vi "5子棋.vi"() -> ()   [LabVIEW 2014]
uses:
  <vilib>/Utility/miscctls.llb/LVPositionTypeDef.ctl
panel:
  out "Black":bool[][](array[boolean])
  out "White":bool[][](array[boolean])
  in  "新遊戲":bool
  out "步數":i32
  in  "結束":bool
  out "悔棋":bool
  out "black control":bool[][](array[boolean])
  out "white control":bool[][](array[boolean])
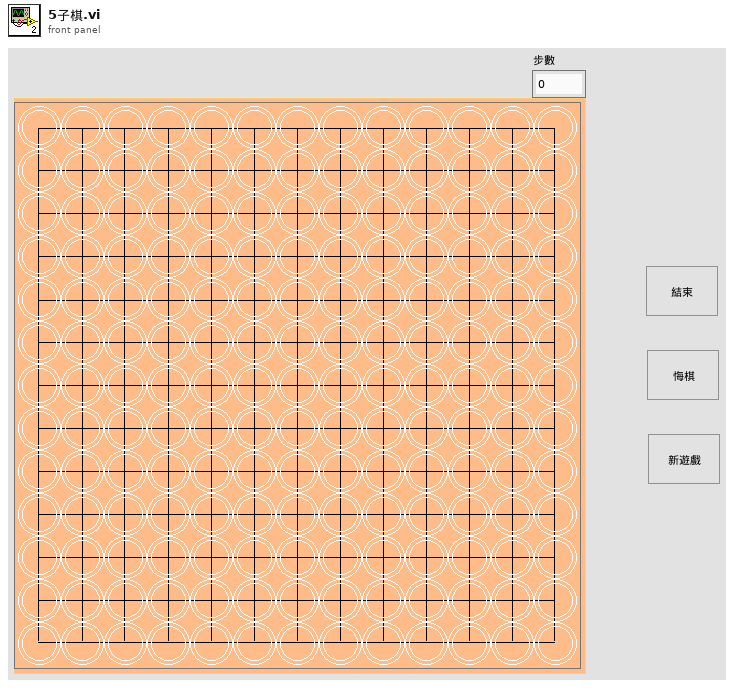
[diagram p1: front panel]
types:
  T1 = typedef "LVPositionTypeDef.ctl" = cluster{"Left":i32, "Top":i32}
  T2 = typedef "LVPoint32TypeDef.ctl" = cluster{"Horizontal":i32, "Vertical":i32}
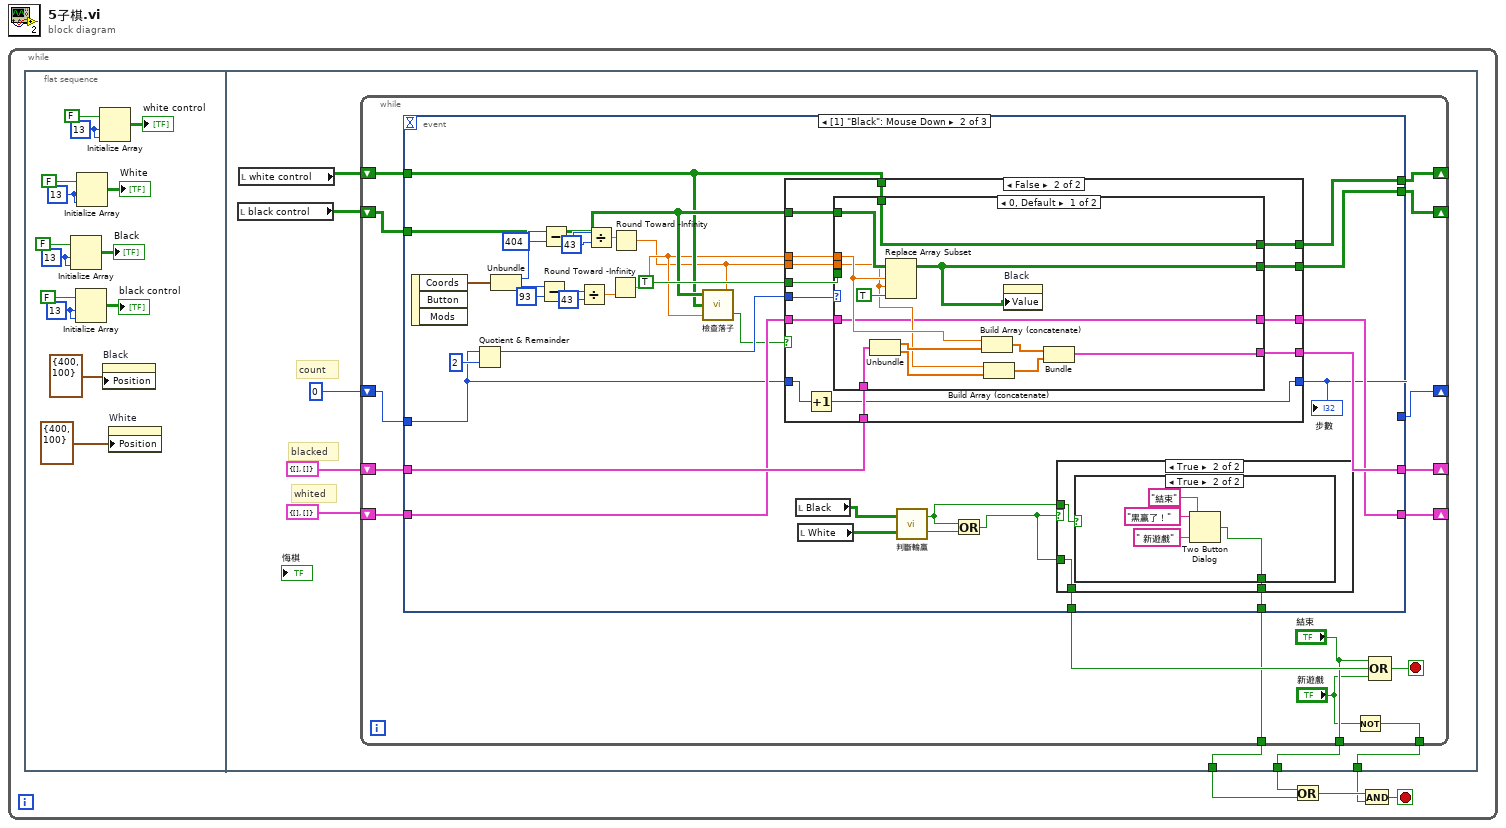
[diagram p0: block diagram]
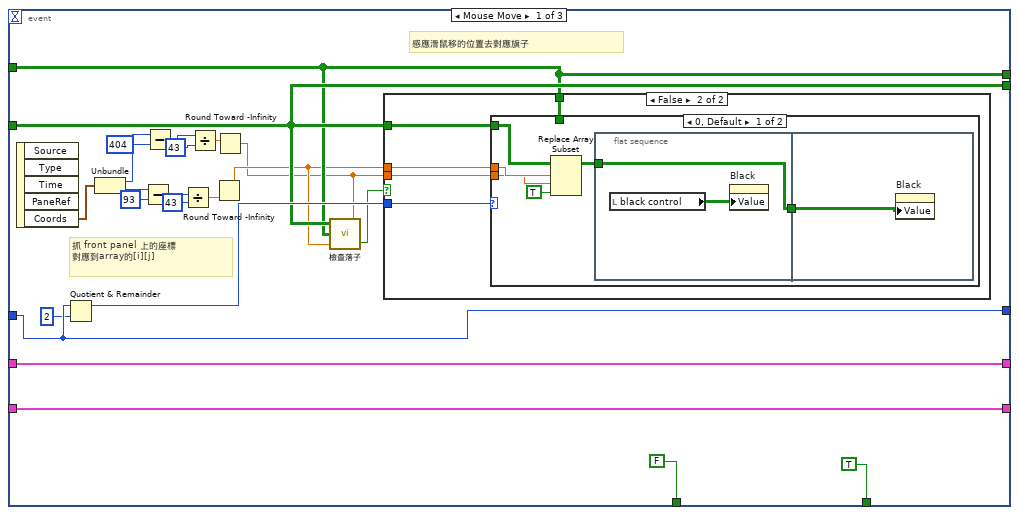
[diagram p2: hidden frame]
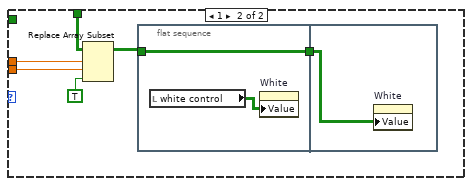
[diagram p4: hidden frame]
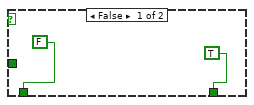
[diagram p5: hidden frame]
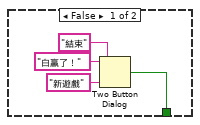
[diagram p6: hidden frame]
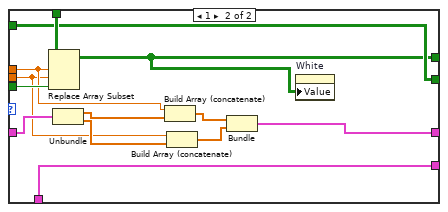
[diagram p8: hidden frame]
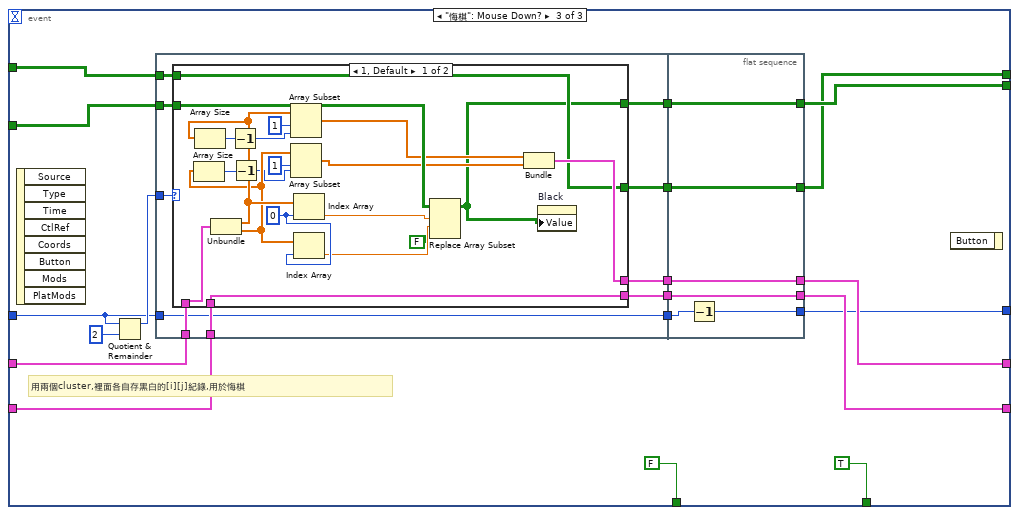
[diagram p9: hidden frame]
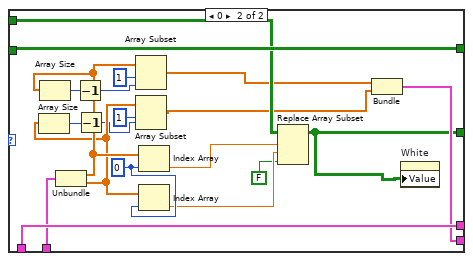
[diagram p10: hidden frame]
diagram:
  n1 = while {
    stop <- w2 stop-if-true
    n2 = flat-sequence {
      tunnel: [w22] -> w4
      tunnel: [w21] -> w5
      tunnel: [w20] -> w1
      frame #0 {
        w17 = 13 ("dimension size")
        w15 = 13 ("dimension size")
        w13 = 13 ("dimension size")
        w11 = 13 ("dimension size")
        n3 = Initialize Array(FALSE, w11, w11) -> (→"Black":bool[][])
        n4 = Initialize Array(FALSE, w17, w17) -> (→"black control":bool[][])
        n5 = Initialize Array(FALSE, w13, w13) -> (→"White":bool[][])
        n6 = Initialize Array(FALSE, w15, w15) -> (→"white control":bool[][])
        n7 = property on="Black" class="Arr (strict)"("Position"=T1 {"Left"=400, "Top"=100}) -> ()  [unwired: 2 in, 2 out]
        n8 = property on="White" class="Arr (strict)"("Position"=T1 {"Left"=400, "Top"=100}) -> ()  [unwired: 2 in, 2 out]
      }
      frame #1 {
        # "count"
        # "whited"
        # "blacked"
        n9 = local read "black control"() -> (w25:bool[][])
        n10 = local read "white control"() -> (w26:bool[][])
        n11 = while {
          shift-right: [w42] -> _
          shift-left: w26 -> [w43]
          shift-right: [w34] -> _
          shift-left: 0 -> [w41]
          shift-right: [w39] -> _
          shift-left: w25 -> [w40]
          shift-right: [w37] -> _
          shift-left: cluster{i32[], i32[]} {[], []} -> [w38]
          shift-right: [w35] -> _
          shift-left: cluster{i32[], i32[]} {[], []} -> [w36]
          tunnel: [w31] -> w22
          tunnel: ["結束"] -> w21
          tunnel: [w28] -> w20
          stop <- w33 stop-if-true
          n12 = event shown="[1] \"Black\": Mouse Down" {
            selector: _ -> [_ _ _]
            dyn-events: _ -> [_ _ _]
            timeout: _ -> [_ _ _]
            tunnel: w43 -> [w49 w102 w192]
            tunnel: [w49 w111 w191] -> w42
            tunnel: w41 -> [w55 w98 w185]
            tunnel: [w55 w97 w184] -> w34
            tunnel: w40 -> [w50 w103 w195]
            tunnel: [w50 w109 w194] -> w39
            tunnel: w38 -> [w53 w108 w198]
            tunnel: [w53 w107 w193] -> w37
            tunnel: w36 -> [w52 w106 w197]
            tunnel: [w52 w105 w196] -> w35
            tunnel: [TRUE w92 TRUE] -> w31
            tunnel: [FALSE w90 FALSE] -> w32
            event Mouse Move {
              # "感應滑鼠移的位置去對應旗子"
              # "抓 front panel 上的座標\n對應到array的[i][j]"
              n13 = event-data() -> ("Coords"=w66:T2)  [unwired: 1 in, 4 out]
              n14 = Quotient & Remainder(x=w55, y=2) -> (x-y*floor(x/y)=w51:i32)  [unwired: 1 out]
              n15 = Unbundle(w66) -> ("Horizontal"=w65:i32, "Vertical"=w61:i32)
              n16 = Subtract(x=w61, y=93) -> (x-y=w59:i32)
              n17 = Subtract(x=w65, y=404) -> (x-y=w63:i32)
              n18 = Divide(x=w59, y=43) -> (x/y=w56:dbl)
              n19 = Divide(x=w63, y=43) -> (x/y=w57:dbl)
              n20 = Round Toward -Infinity(1:w56) -> (0:w48:dbl)
              n21 = Round Toward -Infinity(1:w57) -> (0:w47:dbl)
              n22 = call "檢查落子.vi"("Numeric 2"=w47, "Numeric"=w48, "フ"=w49, "黑"=w50) -> ("黑 or 白？"=w46:bool)
              n23 = case shown="False" w46 {
                tunnel: w47 -> [_ w71]
                tunnel: w48 -> [_ w70]
                tunnel: w49 -> [_ w69]
                tunnel: w50 -> [_ w68]
                tunnel: w51 -> [_ w67]
                frame True {
                }
                frame False {
                  n24 = case shown="0, Default" w67 {
                    tunnel: w71 -> [w72 w83]
                    tunnel: w70 -> [w73 w82]
                    tunnel: w69 -> [_ w81]
                    tunnel: w68 -> [w77 _]
                    frame 0, Default {
                      n25 = Replace Array Subset(array=w77, new element=TRUE ("new element/subarray"), index (row)=w73, index (col)=w72) -> (w75:bool[][])
                      n26 = flat-sequence {
                        tunnel: w75 -> [w79]
                        tunnel: [w79] -> w74
                        tunnel: w74 -> [w80]
                        frame #0 {
                          n27 = local read "black control"() -> (w78:bool[][])
                          n28 = property on="Black" class="Arr (strict)"("Value"=w78) -> ()  [unwired: 2 in, 2 out]
                        }
                        frame #1 {
                          n29 = property on="Black" class="Arr (strict)"("Value"=w80) -> ()  [unwired: 2 in, 2 out]
                        }
                      }
                    }
                    frame 1 {
                      n30 = Replace Array Subset(array=w81, new element=TRUE ("new element/subarray"), index (row)=w82, index (col)=w83) -> (w85:bool[][])
                      n31 = flat-sequence {
                        tunnel: w85 -> [w88]
                        tunnel: [w88] -> w86
                        tunnel: w86 -> [w89]
                        frame #0 {
                          n32 = local read "white control"() -> (w87:bool[][])
                          n33 = property on="White" class="Arr (strict)"("Value"=w87) -> ()  [unwired: 2 in, 2 out]
                        }
                        frame #1 {
                          n34 = property on="White" class="Arr (strict)"("Value"=w89) -> ()  [unwired: 2 in, 2 out]
                        }
                      }
                    }
                  }
                }
              }
            }
            event "Black": Mouse Down {
              n35 = event-data() -> ("Coords"=w113:T2)  [unwired: 1 in, 2 out]
              n36 = Quotient & Remainder(x=w98, y=2) -> (x-y*floor(x/y)=w104:i32)  [unwired: 1 out]
              n37 = Unbundle(w113) -> ("Horizontal"=w123:i32, "Vertical"=w119:i32)
              n38 = Subtract(x=w119, y=93) -> (x-y=w117:i32)
              n39 = Subtract(x=w123, y=404) -> (x-y=w121:i32)
              n40 = Divide(x=w117, y=43) -> (x/y=w114:dbl)
              n41 = Divide(x=w121, y=43) -> (x/y=w115:dbl)
              n42 = Round Toward -Infinity(1:w114) -> (0:w101:dbl)
              n43 = Round Toward -Infinity(1:w115) -> (0:w100:dbl)
              n44 = call "檢查落子.vi"("Numeric 2"=w100, "Numeric"=w101, "フ"=w102, "黑"=w103) -> ("黑 or 白？"=w99:bool)
              n45 = case shown="False" w99 {
                tunnel: TRUE ("new element/subarray") -> [_ w155]
                tunnel: w102 -> [w141 w154]
                tunnel: [w141 w153] -> w111
                tunnel: w103 -> [w140 w152]
                tunnel: [w140 w151] -> w109
                tunnel: w101 -> [_ w150]
                tunnel: w100 -> [_ w149]
                tunnel: w108 -> [w139 w148]
                tunnel: [w139 w147] -> w107
                tunnel: w106 -> [w138 w146]
                tunnel: [w138 w145] -> w105
                tunnel: w104 -> [_ w144]
                tunnel: w98 -> [w137 w143]
                tunnel: [w137 w142] -> w97
                frame True {
                }
                frame False {
                  n46 = Increment(x=w143) -> (x+1=w142:i32)
                  n47 = case shown="0, Default" w144 {
                    tunnel: w149 -> [w159 w172]
                    tunnel: w150 -> [w160 w173]
                    tunnel: w155 -> [_ w181]
                    tunnel: w154 -> [w168 w180]
                    tunnel: [w168 w169] -> w153
                    tunnel: w152 -> [w167 w179]
                    tunnel: [w156 w179] -> w151
                    tunnel: w148 -> [w161 w178]
                    tunnel: [w158 w178] -> w147
                    tunnel: w146 -> [w157 w174]
                    tunnel: [w157 w171] -> w145
                    frame 0, Default {
                      n48 = Unbundle(w161) -> (w165:dbl[], w164:dbl[])
                      n49 = Replace Array Subset(array=w167, new element=TRUE ("new element/subarray"), index (row)=w160, index (col)=w159) -> (w156:bool[][])
                      n50 = Build Array (concatenate)(w160, w165) -> (w163:dbl[])
                      n51 = Build Array (concatenate)(w159, w164) -> (w162:dbl[])
                      n52 = property on="Black" class="Arr (strict)"("Value"=w156) -> ()  [unwired: 2 in, 2 out]
                      n53 = Bundle(w163, w162) -> (w158:cluster{dbl[], dbl[]})  [unwired: 1 in]
                    }
                    frame 1 {
                      n54 = Replace Array Subset(array=w180, new element=w181, index (row)=w173, index (col)=w172) -> (w169:bool[][])
                      n55 = Unbundle(w174) -> (w177:dbl[], w176:dbl[])
                      n56 = Build Array (concatenate)(w173, w177) -> (w170:dbl[])
                      n57 = Build Array (concatenate)(w172, w176) -> (w175:dbl[])
                      n58 = Bundle(w170, w175) -> (w171:cluster{dbl[], dbl[]})  [unwired: 1 in]
                      n59 = property on="White" class="Arr (strict)"("Value"=w169) -> ()  [unwired: 2 in, 2 out]
                    }
                  }
                }
              }
              "步數" <- w97
              n60 = local read "Black"() -> (w93:bool[][])
              n61 = local read "White"() -> (w94:bool[][])
              n62 = call "判斷輸贏.vi"("フ"=w94, "黑"=w93) -> ("フ墓"=w95:bool, "黑贏"=w96:bool)
              n63 = Or(x=w96, y=w95) -> (x .or. y?=w91:bool)
              n64 = case shown="True" w91 {
                tunnel: w96 -> [_ w128]
                tunnel: [TRUE w127] -> w92
                tunnel: w91 -> [_ w126]
                tunnel: [FALSE w126] -> w90
                frame False {
                }
                frame True {
                  n65 = case shown="True" w128 {
                    tunnel: [w129 w133] -> w127
                    frame False {
                      n66 = Two Button Dialog(message="白贏了！", 1:"新遊戲" ("F button name (\"Cancel\")"), 2:"結束" ("T button name (\"OK\")")) -> (T button?=w129:bool)
                    }
                    frame True {
                      n67 = Two Button Dialog(message="黑贏了！", 1:" 新遊戲" ("F button name (\"Cancel\")"), 2:"結束" ("T button name (\"OK\")")) -> (T button?=w133:bool)
                    }
                  }
                }
              }
            }
            event "悔棋": Mouse Down? {
              # "用兩個cluster,裡面各自存黑白的[i][j]紀錄,用於悔棋"
              n68 = event-data() -> ()  [unwired: 1 in, 8 out]
              n69 = Quotient & Remainder(x=w185, y=2) -> (x-y*floor(x/y)=w199:i32)  [unwired: 1 out]
              n70 = flat-sequence {
                tunnel: w199 -> [w210]
                tunnel: w198 -> [w209]
                tunnel: w197 -> [w208]
                tunnel: w195 -> [w206]
                tunnel: w192 -> [w203]
                tunnel: [w207] -> w190
                tunnel: [w205] -> w189
                tunnel: [w204] -> w188
                tunnel: [w202] -> w187
                tunnel: [w201] -> w186
                tunnel: w185 -> [w201]
                tunnel: [w253] -> w191
                tunnel: [w254] -> w193
                tunnel: [w255] -> w194
                tunnel: [w256] -> w196
                tunnel: w190 -> [w256]
                tunnel: w189 -> [w255]
                tunnel: w188 -> [w254]
                tunnel: w187 -> [w253]
                tunnel: w186 -> [w252]
                tunnel: [w251] -> w184
                frame #0 {
                  n71 = case shown="1, Default" w210 {
                    tunnel: w209 -> [w217 w249]
                    tunnel: w208 -> [w230 w248]
                    tunnel: [w230 w246] -> w207
                    tunnel: w206 -> [w229 w250]
                    tunnel: [w211 w250] -> w205
                    tunnel: [w228 w249] -> w204
                    tunnel: w203 -> [w227 w247]
                    tunnel: [w227 w231] -> w202
                    frame 1, Default {
                      w226 = 0 ("index")
                      n72 = Unbundle(w217) -> (w223:dbl[], w220:dbl[])
                      n73 = Array Size(array=w220) -> (size(s)=w219:i32)
                      n74 = Array Size(array=w223) -> (size(s)=w222:i32)
                      n75 = Decrement(x=w222) -> (x-1=w221:i32)
                      n76 = Decrement(x=w219) -> (x-1=w218:i32)
                      n77 = Array Subset(array=w223, index=1, length=w221) -> (w216:dbl[])
                      n78 = Array Subset(array=w220, index=1, length=w218) -> (w215:dbl[])
                      n79 = Index Array(array=w223, index=w226) -> (element=w214:dbl)
                      n80 = Index Array(array=w220, index=w226) -> (element=w213:dbl)
                      n81 = Replace Array Subset(array=w229, new element=FALSE ("new element/subarray"), index (row)=w214, index (col)=w213) -> (w211:bool[][])
                      n82 = Bundle(w216, w215) -> (w228:cluster{dbl[], dbl[]})  [unwired: 1 in]
                      n83 = property on="Black" class="Arr (strict)"("Value"=w211) -> ()  [unwired: 2 in, 2 out]
                    }
                    frame 0 {
                      w245 = 0 ("index")
                      n84 = Unbundle(w248) -> (w239:dbl[], w236:dbl[])
                      n85 = Array Size(array=w236) -> (size(s)=w235:i32)
                      n86 = Array Size(array=w239) -> (size(s)=w238:i32)
                      n87 = Decrement(x=w238) -> (x-1=w237:i32)
                      n88 = Decrement(x=w235) -> (x-1=w234:i32)
                      n89 = Array Subset(array=w239, index=1, length=w237) -> (w233:dbl[])
                      n90 = Array Subset(array=w236, index=1, length=w234) -> (w232:dbl[])
                      n91 = Index Array(array=w239, index=w245) -> (element=w244:dbl)
                      n92 = Index Array(array=w236, index=w245) -> (element=w243:dbl)
                      n93 = Replace Array Subset(array=w247, new element=FALSE ("new element/subarray"), index (row)=w244, index (col)=w243) -> (w231:bool[][])
                      n94 = Bundle(w233, w232) -> (w246:cluster{dbl[], dbl[]})  [unwired: 1 in]
                      n95 = property on="White" class="Arr (strict)"("Value"=w231) -> ()  [unwired: 2 in, 2 out]
                    }
                  }
                }
                frame #1 {
                  n96 = Decrement(x=w252) -> (x-1=w251:i32)
                }
              }
              n97 = event-data() -> ()  [unwired: 2 in, 1 out]
            }
          }
          n98 = Not(x="新遊戲") -> (.not. x?=w28:bool)
          n99 = Compound Arithmetic op=OR("結束", w32, "新遊戲") -> (w33:bool)
        }
      }
    }
    n100 = Or(x=w5, y=w4) -> (x .or. y?=w3:bool)
    n101 = And(x=w3, y=w1) -> (x .and. y?=w2:bool)
  }
